vi "Errorbar1002.vi"   [LabVIEW 2013]
uses:
  <vilib>/Heliosphere Research LLC/Advanced Plotting Toolkit/api_plotting/ErrorbarProperties.ctl
  <vilib>/Heliosphere Research LLC/Advanced Plotting Toolkit/typedefs/PlotColor.ctl
  <vilib>/Heliosphere Research LLC/Advanced Plotting Toolkit/properties/Display.ctl
  <vilib>/Heliosphere Research LLC/Advanced Plotting Toolkit/Advanced Plotting Toolkit.lvlib
types:
  T1 = typedef "Advanced Plotting Toolkit.lvlib/PlotColor.ctl" = u32
  T2 = typedef "Advanced Plotting Toolkit.lvlib/ErrorbarProperties.ctl" = cluster{"Color":T1, "Line Width":dbl, "Cap Size":dbl, "Display":T3}
  T3 = typedef "Advanced Plotting Toolkit.lvlib/Display.ctl" = cluster{"Alpha":dbl, "Z Order":dbl}
  T4 = typedef "Advanced Plotting Toolkit.lvlib/PlotID.ctl" = i32
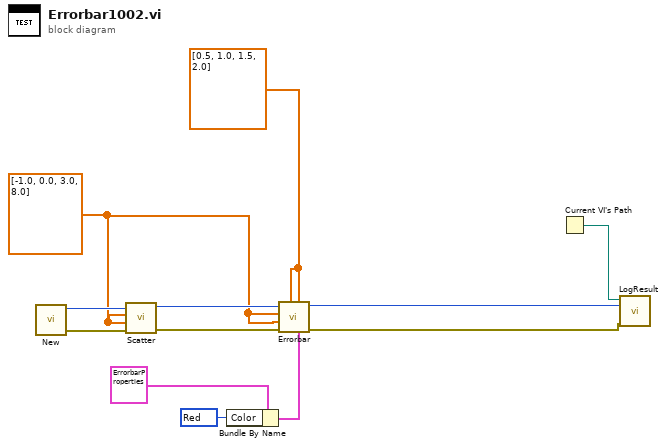
[diagram p0: block diagram]
diagram:
  w1 = T1 16711680 items=["Automatic"=2147483647, "Black"=0, "White"=16777215, "Red"=16711680, "Green"=2263842, "Blue"=255, "Cyan"=65535, "Magenta"=16711935, "Yellow"=16776960] ("Color")
  w4 = dbl[] [0.5, 1.0, 1.5, 2.0] ("X Errors")
  w5 = dbl[] [-1.0, 0.0, 3.0, 8.0] ("X Data")
  n1 = call <vilib>:"New.vi"() -> ("error out"=w6:errorcluster, "Plot ID"=w9:T4)  [unwired: 10 in]
  n2 = call <vilib>:"Scatter.vi"("error in (no error)"=w6, "Y Data"=w5, "X Data"=w5, "Plot ID"=w9) -> ("error out"=w7:errorcluster, "Plot ID Out"=w8:T4)  [unwired: 6 in]
  n3 = Bundle By Name(cluster=T2 {"Color"=2147483647, "Line Width"=nan, "Cap Size"=nan, "Display"={"Alpha"=nan, "Z Order"=nan}} ("Errorbar Properties"), "Color"=w1) -> (w2:T2)
  n4 = call <vilib>:"Errorbar.vi"("Properties"=w2, "Y Errors"=w4, "X Errors"=w4, "error in (no error)"=w7, "Y Data"=w5, "X Data"=w5, "Plot ID"=w8) -> ("error out"=w10:errorcluster, "Plot ID out"=w11:T4)  [unwired: 3 in]
  n5 = Current VI's Path() -> (path=w12:path)
  n6 = call "LogResult.vi"("Test Result"=w10, "Test Artifact"=w11, "VI Path"=w12) -> ()  [unwired: 9 in]
